vi "EMG_Control_State_Machine.vi"(0 "Biceps hardly contracted?":bool, 1 "Biceps second threshold (V)":dbl, 2 "Biceps mean amplitude (V)":dbl, 3 "Biceps max amplitude (V)":dbl, 5 "Biceps contracted?":bool, 9 "Triceps contracted?":bool, 11 "Triceps hardly contracted?":bool, 12 "Triceps second threshold (V)":dbl, 13 "Triceps mean amplitude (V)":dbl, 14 "Triceps max amplitude (V)":dbl) -> (4 "EMG Control":T1(ring), 10 "EMG signal max amplitude (V)":dbl, 15 "EMG signal mean amplitude (V)":dbl)   [LabVIEW 2015]
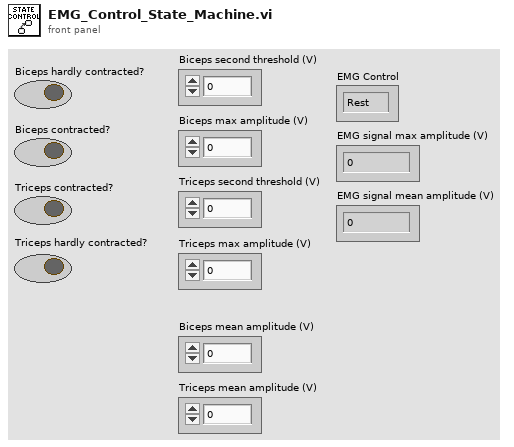
[diagram p1: front panel]
types:
  T1 = enum16{"Rest", "Triceps hardly contracted", "Triceps contracted", "Biceps hardly contracted", "Biceps contracted", "Change mode"}
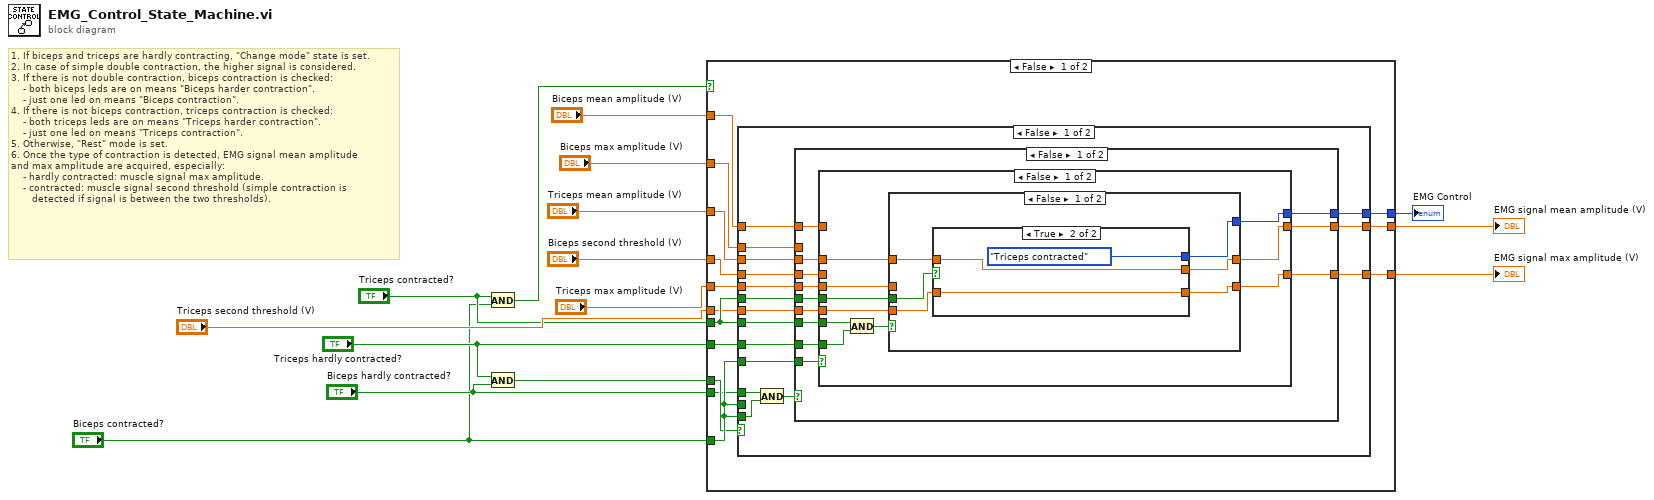
[diagram p0: block diagram]
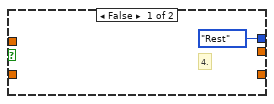
[diagram p2: hidden frame]
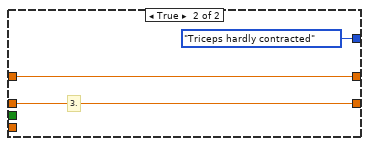
[diagram p3: hidden frame]
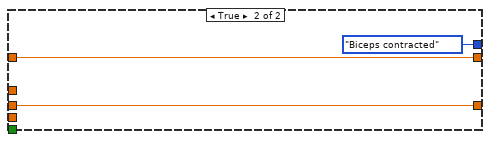
[diagram p4: hidden frame]
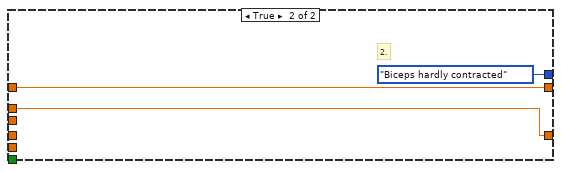
[diagram p5: hidden frame]
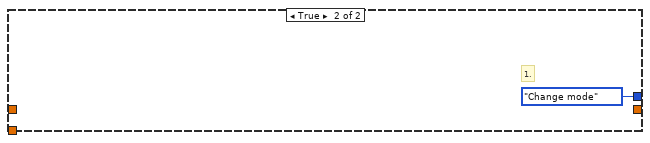
[diagram p6: hidden frame]
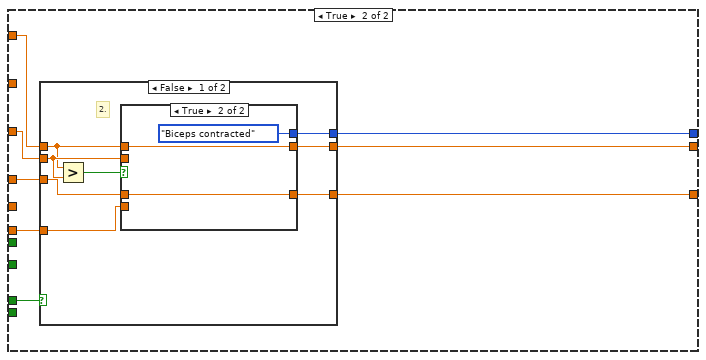
[diagram p7: hidden frame]
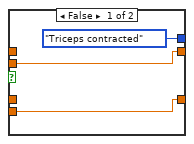
[diagram p8: hidden frame]
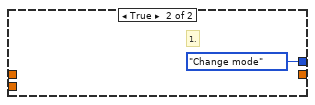
[diagram p9: hidden frame]
diagram:
  # "1. If biceps and triceps are hardly contracting, \"Change mode\" state is set.\n2. In case of simple double contraction, the higher signal is considered.\n3. If there is not double contraction, biceps contraction is checked:\n    - both biceps leds are on means \"Biceps harder contraction\".\n    - just one led on means \"Biceps contraction\".\n4. If there is not biceps contraction, triceps contraction is checked:\n    - both triceps leds are on means \"Triceps harder contraction\".\n    - just one led on means \"Triceps contraction\".\n5. Otherwise, \"Rest\" mode is set.\n6. Once the type of contraction is detected, EMG signal mean amplitude\nand max amplitude are acquired, especially:\n    - hardly contracted: muscle signal max amplitude.\n    - contracted: muscle signal second threshold (simple contraction is\n       detected if signal is between the two thresholds)."
  n1 = And(x="Triceps contracted?", y="Biceps contracted?") -> (x .and. y?=w1:bool)
  n2 = And(x="Triceps hardly contracted?", y="Biceps hardly contracted?") -> (x .and. y?=w15:bool)
  n3 = case shown="False" w1 {
    tunnel: "Triceps contracted?" -> [w29 _]
    tunnel: "Biceps contracted?" -> [w28 _]
    tunnel: w15 -> [w27 w88]
    tunnel: [w26 w95] -> w14
    tunnel: "Triceps second threshold (V)" -> [w25 w92]
    tunnel: [w24 w91] -> w12
    tunnel: "Triceps mean amplitude (V)" -> [w23 w94]
    tunnel: [w22 w93] -> w10
    tunnel: "Triceps max amplitude (V)" -> [w21 _]
    tunnel: "Biceps mean amplitude (V)" -> [w20 w89]
    tunnel: "Biceps second threshold (V)" -> [w19 w90]
    tunnel: "Biceps max amplitude (V)" -> [w18 _]
    tunnel: "Triceps hardly contracted?" -> [w17 _]
    tunnel: "Biceps hardly contracted?" -> [w16 _]
    frame False {
      n4 = case shown="False" w27 {
        tunnel: w16 -> [w45 _]
        tunnel: w28 -> [w44 _]
        tunnel: w28 -> [_ _]
        tunnel: w28 -> [w42 _]
        tunnel: w29 -> [w41 _]
        tunnel: w17 -> [w40 _]
        tunnel: w29 -> [w39 _]
        tunnel: [w38 T1."Change mode"] -> w26
        tunnel: w25 -> [w37 _]
        tunnel: [w36 _] -> w24
        tunnel: w23 -> [w35 _]
        tunnel: [w34 _] -> w22
        tunnel: w21 -> [w33 _]
        tunnel: w20 -> [w32 _]
        tunnel: w19 -> [w31 _]
        tunnel: w18 -> [w30 _]
        frame False {
          n5 = And(x=w45, y=w44) -> (x .and. y?=w43:bool)
          n6 = case shown="False" w43 {
            tunnel: [w56 T1."Biceps hardly contracted"] -> w38
            tunnel: w42 -> [w57 _]
            tunnel: w41 -> [w55 _]
            tunnel: w40 -> [w54 _]
            tunnel: w39 -> [w53 _]
            tunnel: w37 -> [w52 _]
            tunnel: [w51 w85] -> w36
            tunnel: w35 -> [w50 _]
            tunnel: [w49 w84] -> w34
            tunnel: w33 -> [w48 _]
            tunnel: w32 -> [w47 w84]
            tunnel: w31 -> [w46 _]
            tunnel: w30 -> [_ w85]
            frame False {
              n7 = case shown="False" w57 {
                tunnel: [w64 T1."Biceps contracted"] -> w56
                tunnel: w55 -> [w67 _]
                tunnel: w54 -> [w66 _]
                tunnel: w53 -> [w63 _]
                tunnel: w52 -> [w62 _]
                tunnel: [w61 w81] -> w51
                tunnel: w50 -> [w60 _]
                tunnel: [w59 w82] -> w49
                tunnel: w48 -> [w58 _]
                tunnel: w47 -> [_ w82]
                tunnel: w46 -> [_ w81]
                frame False {
                  n8 = And(x=w67, y=w66) -> (x .and. y?=w65:bool)
                  n9 = case shown="False" w65 {
                    tunnel: [w72 T1."Triceps hardly contracted"] -> w64
                    tunnel: w63 -> [w73 _]
                    tunnel: w62 -> [w71 _]
                    tunnel: [w70 w78] -> w61
                    tunnel: w60 -> [w69 w79]
                    tunnel: [w68 w79] -> w59
                    tunnel: w58 -> [_ w78]
                    frame False {
                      n10 = case shown="True" w73 {
                        tunnel: [T1."Rest" T1."Triceps contracted"] -> w72
                        tunnel: w71 -> [_ w76]
                        tunnel: [_ w76] -> w70
                        tunnel: w69 -> [_ w75]
                        tunnel: [_ w75] -> w68
                        frame False {
                          # "4."
                        }
                        frame True {
                        }
                      }
                    }
                    frame True {
                      # "3."
                    }
                  }
                }
                frame True {
                }
              }
            }
            frame True {
              # "2."
            }
          }
        }
        frame True {
          # "1."
        }
      }
    }
    frame True {
      n11 = case shown="False" w88 {
        tunnel: [w102 T1."Change mode"] -> w95
        tunnel: w94 -> [w101 _]
        tunnel: [w100 _] -> w93
        tunnel: w92 -> [w99 _]
        tunnel: [w98 _] -> w91
        tunnel: w90 -> [w97 _]
        tunnel: w89 -> [w96 _]
        frame False {
          # "2."
          n12 = Greater?(x=w96, y=w101) -> (0:w103:bool)
          n13 = case shown="True" w103 {
            tunnel: [T1."Triceps contracted" T1."Biceps contracted"] -> w102
            tunnel: [w105 w107] -> w100
            tunnel: w101 -> [w105 _]
            tunnel: w99 -> [w104 _]
            tunnel: [w104 w108] -> w98
            tunnel: w97 -> [_ w108]
            tunnel: w96 -> [_ w107]
            frame False {
            }
            frame True {
            }
          }
        }
        frame True {
          # "1."
        }
      }
    }
  }
  "EMG Control" <- w14
  "EMG signal max amplitude (V)" <- w12
  "EMG signal mean amplitude (V)" <- w10
